vi "StopMonitFGV.vi"(10 "Command":enum16{"Write", "Read"}(ring), 11 "IN":bool) -> (3 "OUT":bool)   [LabVIEW 2015]
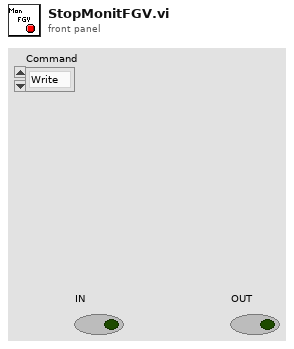
[diagram p1: front panel]
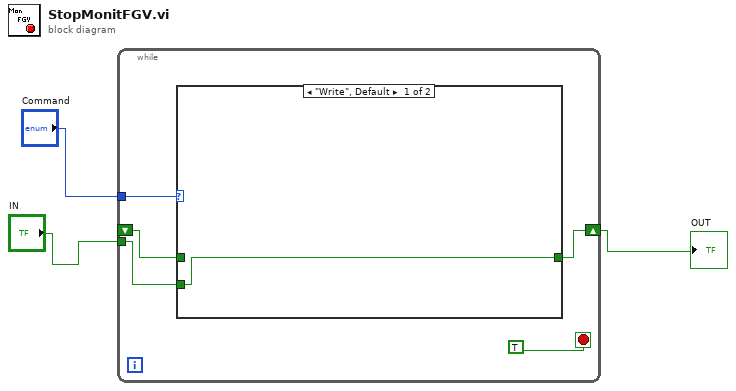
[diagram p0: block diagram]
diagram:
  n1 = while {
    tunnel: "Command" -> [w8]
    shift-right: [w7] -> w1
    shift-left: _ -> [w4]
    tunnel: "IN" -> [w5]
    stop <- TRUE stop-if-true
    n2 = case shown="\"Write\", Default" w8 {
      tunnel: [w9 w10] -> w7
      tunnel: w5 -> [w9 _]
      tunnel: w4 -> [_ w10]
      frame "Write", Default {
      }
      frame "Read" {
      }
    }
  }
  "OUT" <- w1
